vi "Run.vi"(8 "error in (no error)":errorcluster caption="entrée d'erreur (pas d'erreur)", 9 "probas_pred":string[][](array[string]), 10 "y_true":string[][](array[string]), 11 "Precision_Recall_Curve.lvclass":refnum<class "Precision_Recall_Curve.lvclass">) -> (0 "error out":errorcluster caption="sortie d'erreur", 2 "Data":T1, 3 "Precision_Recall_Curve.lvclass":refnum<class "Precision_Recall_Curve.lvclass">)   [LabVIEW 2020, in "Precision_Recall_Curve.lvclass"]
doc: "Returns :\n\n- precision : array, shape = [n_thresholds + 1]\nPrecision values such that element i is the precision of predictions with score >= thresholds[i] and the last element is 1.\n\n- recall : array, shape = [n_thresholds + 1]\nDecreasing recall values such that element i is the recall of predictions with score >= thresholds[i] and the last element is 0.\n\n- thresholds : array, shape = [n_thresholds <= len(np.unique(probas_pred))]\nIncreasing thresholds on the decision function used to compute precision and recall."
uses:
  Precision_Recall_Curve.lvclass
  Precision_Recall_Curve.lvclass/Precision_Recall_Curve.ctl
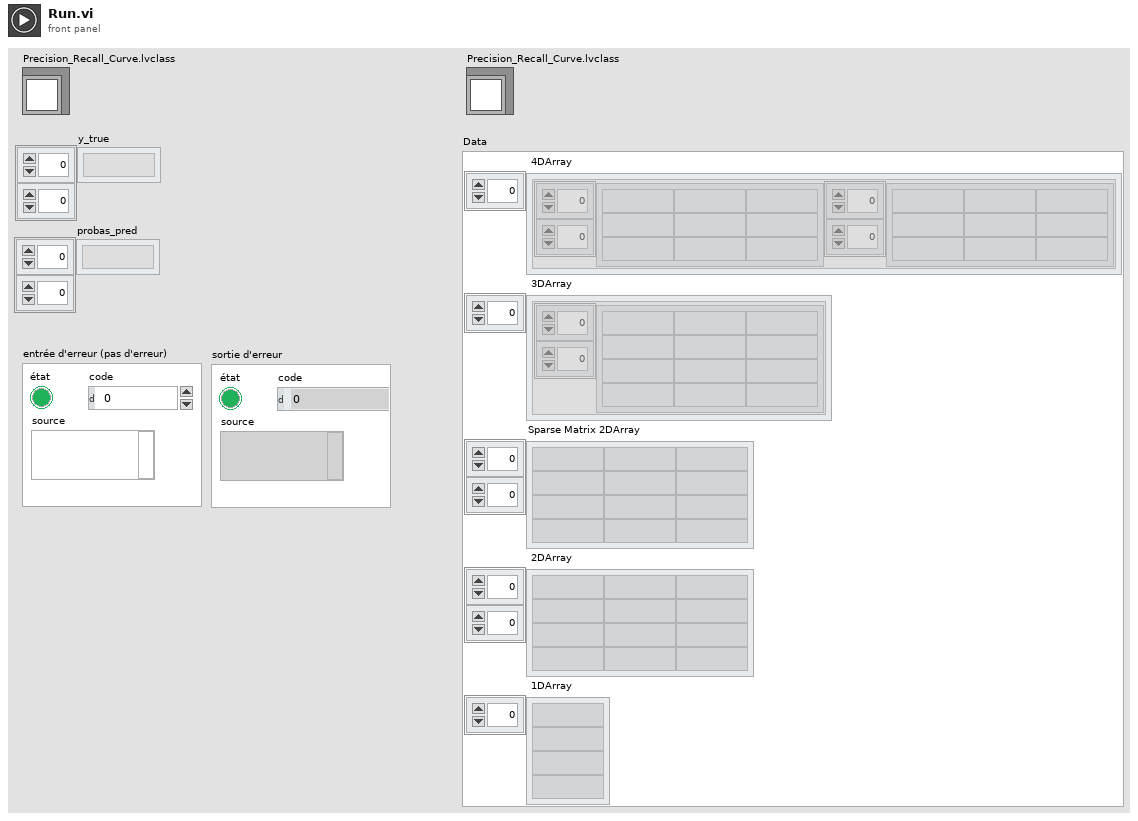
[diagram p1: front panel]
types:
  T1 = cluster{" 4DArray":cluster{"1":string[][], "2":string[][]}[], " 3DArray":cluster{"Tableau":string[][]}[], "Sparse Matrix 2DArray":string[][], " 2DArray":string[][], " 1DArray":string[]}
  T2 = cluster{"dtype_pos_label":string, "pos_label":string}
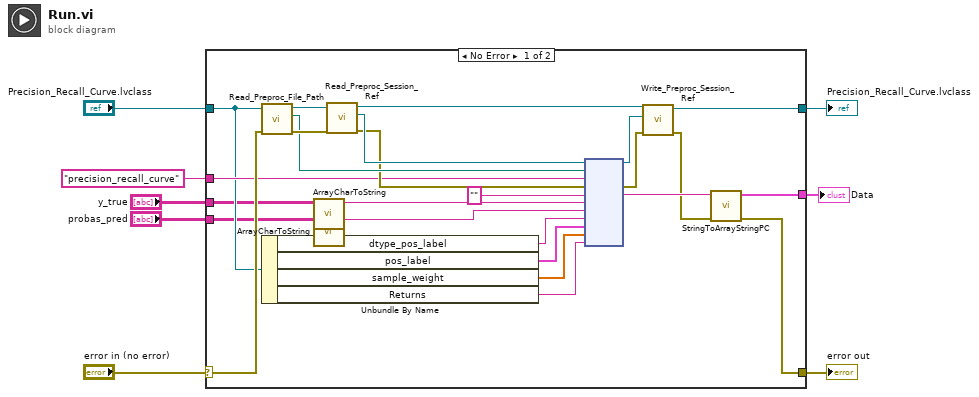
[diagram p0: block diagram]
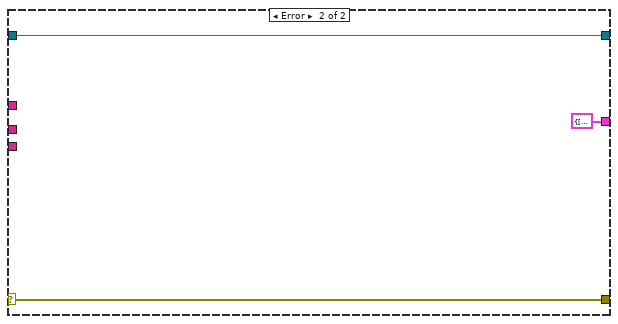
[diagram p2: hidden frame]
diagram:
  n1 = case shown="No Error" "error in (no error)" {
    selector: "error in (no error)" -> [w24 w36]
    tunnel: [w9 w36] -> w7
    tunnel: [w13 w35] -> w5
    tunnel: "Precision_Recall_Curve.lvclass" -> [w22 w35]
    tunnel: "precision_recall_curve" -> [w23 _]
    tunnel: "y_true" -> [w17 _]
    tunnel: "probas_pred" -> [w16 _]
    tunnel: [w10 T1 {" 4DArray"=[], " 3DArray"=[], "Sparse Matrix 2DArray"=[], " 2DArray"=[], " 1DArray"=[]} ("Data")] -> w1
    frame No Error {
      n2 = call-dynamic "Read_Preproc_File_Path.vi"("error in (no error)"=w24, "Python in"=w22) -> ("error out"=w32:errorcluster, "File_Path"=w31:path, "Python out"=w33:refnum<class "Precision_Recall_Curve.lvclass">)  [unwired: 7 in]
      n3 = Unbundle By Name(w22) -> ("dtype_pos_label"=w21:string, "pos_label"=w20:T2, "sample_weight"=w19:dbl[], "Returns"=w18:string)
      n4 = call "ArrayCharToString.vi"("TAB"=w17) -> ("Instruction"=w15:string)  [unwired: 10 in]
      n5 = call "ArrayCharToString.vi"("TAB"=w16) -> ("Instruction"=w14:string)  [unwired: 10 in]
      n6 = call-dynamic "Read_Preproc_Session_Ref.vi"("error in (no error)"=w32, "Python in"=w33) -> ("error out"=w29:errorcluster, "Session_ref"=w30:refnum<k35>, "Python out"=w28:refnum<class "Precision_Recall_Curve.lvclass">)  [unwired: 7 in]
      n7 = node(w30, w31, w23, w29, "", w15, w14, w21, w20, w19, w18) -> (w26:refnum<k35>, w27:errorcluster, w12:string)  [unwired: 6 in, 2 out]
      n8 = call-dynamic "Write_Preproc_Session_Ref.vi"("error in (no error)"=w27, "Session_ref"=w26, "Python in"=w28) -> ("error out"=w11:errorcluster, "Python out"=w13:refnum<class "Precision_Recall_Curve.lvclass">)  [unwired: 7 in]
      n9 = call "StringToArrayStringPC.vi"("sortie d'erreur"=w11, "Return value"=w12) -> ("sortie d'erreur"=w9:errorcluster, "Data"=w10:T1)  [unwired: 8 in]
    }
    frame Error {
    }
  }
  "error out" <- w7
  "Precision_Recall_Curve.lvclass" <- w5
  "Data" <- w1
